vi "Check-GUI-values-for-conflicts.vi"(8 "error in (no error)":errorcluster, 11 "Data ref. in":refnum<data-value>) -> (0 "error out":errorcluster, 1 "Passed?":bool, 3 "Data ref.":refnum<data-value>)   [LabVIEW 2013, in "CameraVision.lvlib" / "CV-Main.lvclass"]
uses:
  CV-Main.lvclass
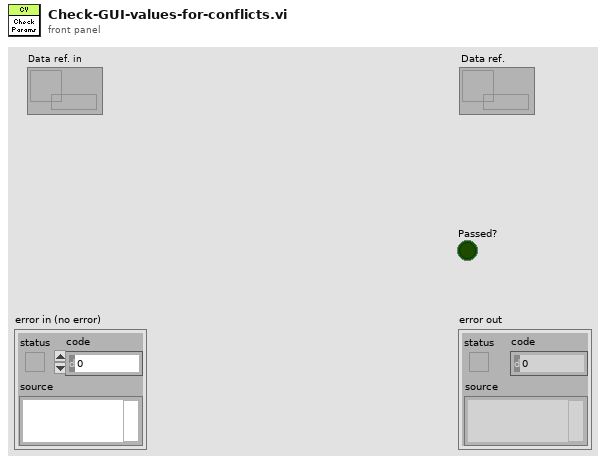
[diagram p1: front panel]
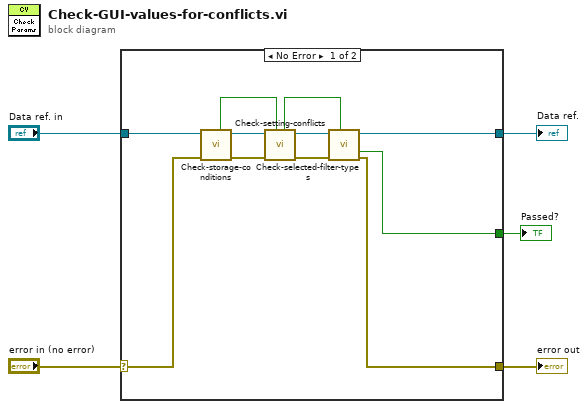
[diagram p0: block diagram]
diagram:
  n1 = case shown="No Error" "error in (no error)" {
    selector: "error in (no error)" -> [w8 w18]
    tunnel: [w7 w18] -> w4
    tunnel: "Data ref. in" -> [w10 w17]
    tunnel: [w6 w17] -> w2
    tunnel: [w9 _] -> w1
    frame No Error {
      n2 = call "Check-storage-conditions.vi"("error in (no error)"=w8, "Data ref. in"=w10) -> ("error out"=w11:errorcluster, "Data ref."=w12:refnum<data-value>, "Passed?"=w13:bool)  [unwired: 7 in]
      n3 = call "Check-setting-conflicts.vi"("Passed? in"=w13, "error in"=w11, "Data ref. in"=w12) -> ("error IO"=w16:errorcluster, "Data ref."=w14:refnum<data-value>, "Passed?"=w15:bool)  [unwired: 6 in]
      n4 = call "Check-selected-filter-types.vi"("Passed? in"=w15, "error in"=w16, "Data ref in"=w14) -> ("error IO"=w7:errorcluster, "Data ref"=w6:refnum<data-value>, "Passed?"=w9:bool)  [unwired: 6 in]
    }
    frame Error {
    }
  }
  "error out" <- w4
  "Data ref." <- w2
  "Passed?" <- w1
